vi "Sensor State.vi"(1 "Input":dbl, 2 "Sensor State FGV Selector":T1, 3 "Action":T2) -> (0 "Output":dbl)   [LabVIEW 2013]
uses:
  Action.ctl
  Sensor State FGV Selector.ctl
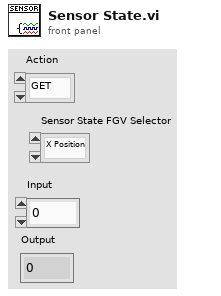
[diagram p1: front panel]
types:
  T1 = typedef "Sensor State FGV Selector.ctl" = enum16{"X Position", "Y Position", "Z Position", "Sum", "Division"}
  T2 = typedef "Action.ctl" = enum16{"GET", "PUT", "DELETE"}
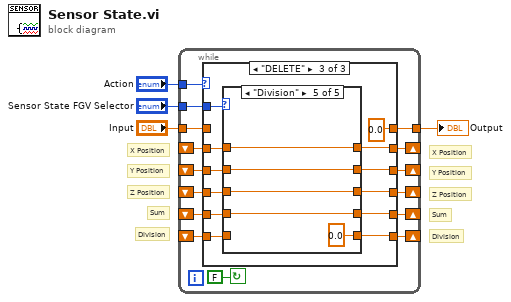
[diagram p0: block diagram]
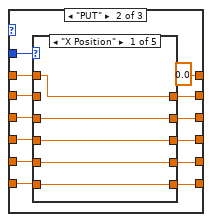
[diagram p7: hidden frame]
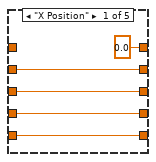
[diagram p12: hidden frame]
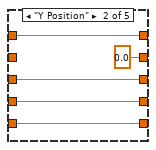
[diagram p13: hidden frame]
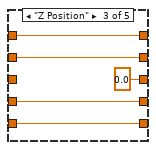
[diagram p14: hidden frame]
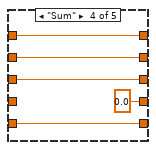
[diagram p15: hidden frame]
diagram:
  # "Division"
  # "Sum"
  # "Z Position"
  # "Y Position"
  # "X Position"
  # "Division"
  # "Sum"
  # "Z Position"
  # "Y Position"
  # "X Position"
  n1 = while {
    tunnel: "Action" -> [w18]
    tunnel: "Sensor State FGV Selector" -> [w17]
    tunnel: "Input" -> [w16]
    tunnel: [w15] -> w1
    shift-right: [w13] -> _
    shift-left: _ -> [w14]
    shift-right: [w11] -> _
    shift-left: _ -> [w12]
    shift-right: [w9] -> _
    shift-left: _ -> [w10]
    shift-right: [w7] -> _
    shift-left: _ -> [w8]
    shift-right: [w5] -> _
    shift-left: _ -> [w6]
    stop <- FALSE continue-if-true
    n2 = case shown="\"DELETE\"" w18 {
      tunnel: w17 -> [w31 w68 w106]
      tunnel: w16 -> [_ w69 _]
      tunnel: [w20 0.0 0.0] -> w15
      tunnel: w14 -> [w30 w67 w105]
      tunnel: [w29 w62 w99] -> w13
      tunnel: w12 -> [w28 w66 w104]
      tunnel: [w27 w61 w98] -> w11
      tunnel: w10 -> [w26 w65 w103]
      tunnel: [w25 w60 w97] -> w9
      tunnel: w8 -> [w24 w64 w102]
      tunnel: [w23 w59 w96] -> w7
      tunnel: w6 -> [w22 w63 w101]
      tunnel: [w21 w58 w95] -> w5
      frame "GET", Default {
        n3 = case shown="\"Division\"" w31 {
          tunnel: [w32 w37 w42 w47 w52] -> w20
          tunnel: w30 -> [w32 w41 w46 w51 w56]
          tunnel: [w32 w41 w46 w51 w56] -> w29
          tunnel: w28 -> [w36 w37 w45 w50 w55]
          tunnel: [w36 w37 w45 w50 w55] -> w27
          tunnel: w26 -> [w35 w40 w42 w49 w54]
          tunnel: [w35 w40 w42 w49 w54] -> w25
          tunnel: w24 -> [w34 w39 w44 w47 w53]
          tunnel: [w34 w39 w44 w47 w53] -> w23
          tunnel: w22 -> [w33 w38 w43 w48 w52]
          tunnel: [w33 w38 w43 w48 w52] -> w21
          frame "X Position" {
          }
          frame "Y Position" {
          }
          frame "Z Position" {
          }
          frame "Sum" {
          }
          frame "Division" {
          }
        }
      }
      frame "PUT" {
        n4 = case shown="\"X Position\"" w68 {
          tunnel: w67 -> [_ w79 w84 w89 w94]
          tunnel: [w70 w79 w84 w89 w94] -> w62
          tunnel: w66 -> [w74 _ w83 w88 w93]
          tunnel: [w74 w75 w83 w88 w93] -> w61
          tunnel: w65 -> [w73 w78 _ w87 w92]
          tunnel: [w73 w78 w80 w87 w92] -> w60
          tunnel: w64 -> [w72 w77 w82 _ w91]
          tunnel: [w72 w77 w82 w85 w91] -> w59
          tunnel: w63 -> [w71 w76 w81 w86 _]
          tunnel: [w71 w76 w81 w86 w90] -> w58
          tunnel: w69 -> [w70 w75 w80 w85 w90]
          frame "X Position" {
          }
          frame "Y Position" {
          }
          frame "Z Position" {
          }
          frame "Sum" {
          }
          frame "Division" {
          }
        }
      }
      frame "DELETE" {
        n5 = case shown="\"Division\"" w106 {
          tunnel: w105 -> [_ w116 w121 w126 w131]
          tunnel: [0.0 ("Input") w116 w121 w126 w131] -> w99
          tunnel: w104 -> [w111 _ w120 w125 w130]
          tunnel: [w111 0.0 ("Input") w120 w125 w130] -> w98
          tunnel: w103 -> [w110 w115 _ w124 w129]
          tunnel: [w110 w115 0.0 ("Input") w124 w129] -> w97
          tunnel: w102 -> [w109 w114 w119 _ w128]
          tunnel: [w109 w114 w119 0.0 ("Input") w128] -> w96
          tunnel: w101 -> [w108 w113 w118 w123 _]
          tunnel: [w108 w113 w118 w123 0.0 ("Input")] -> w95
          frame "X Position" {
          }
          frame "Y Position" {
          }
          frame "Z Position" {
          }
          frame "Sum" {
          }
          frame "Division" {
          }
        }
      }
    }
  }
  "Output" <- w1
